vi "step2 SolveLowerLeftCornerPiece.vi"(8 "error in (no error)":errorcluster, 10 "operation queue":refnum<queue>, 11 "cube in":T1) -> (0 "error out":errorcluster, 2 "operation queue out":refnum<queue>, 3 "cube out":T1)   [LabVIEW 2011]
doc: "Rotate cube as necessary so that the top middle piece matches the desired start colour.\n\nNo transformations are done in this VI, the operations are loaded on the the operation queue bus."
uses:
  Typedef/cube.ctl
  Typedef/face.ctl
  Typedef/main state.ctl
  Typedef/operation.ctl
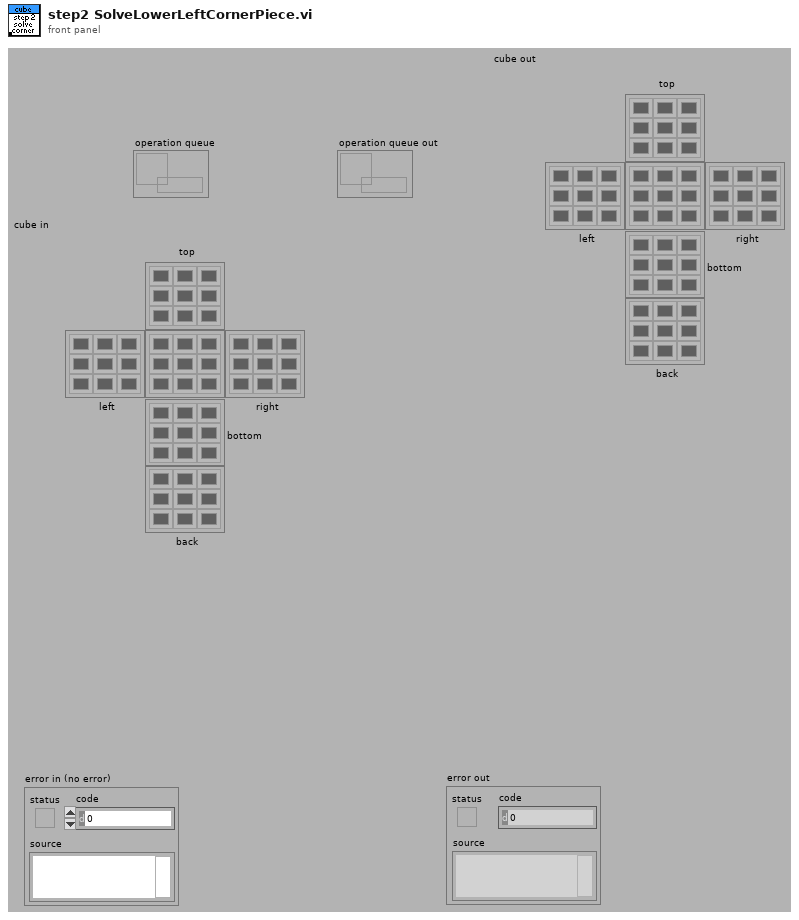
[diagram p1: front panel]
types:
  T1 = typedef "cube.ctl" = cluster{"top":T2, "left":T2, "right":T2, "bottom":T2, "back":T2, "front":T2}
  T2 = typedef "face.ctl" = u32[][]
  T3 = typedef "operation.ctl" = enum16{"nop", "T+", "T-", "F+", "F-", "L+", "L-", "R+", "R-", "B+", "B-", "<--", "-->", "^", "V"}
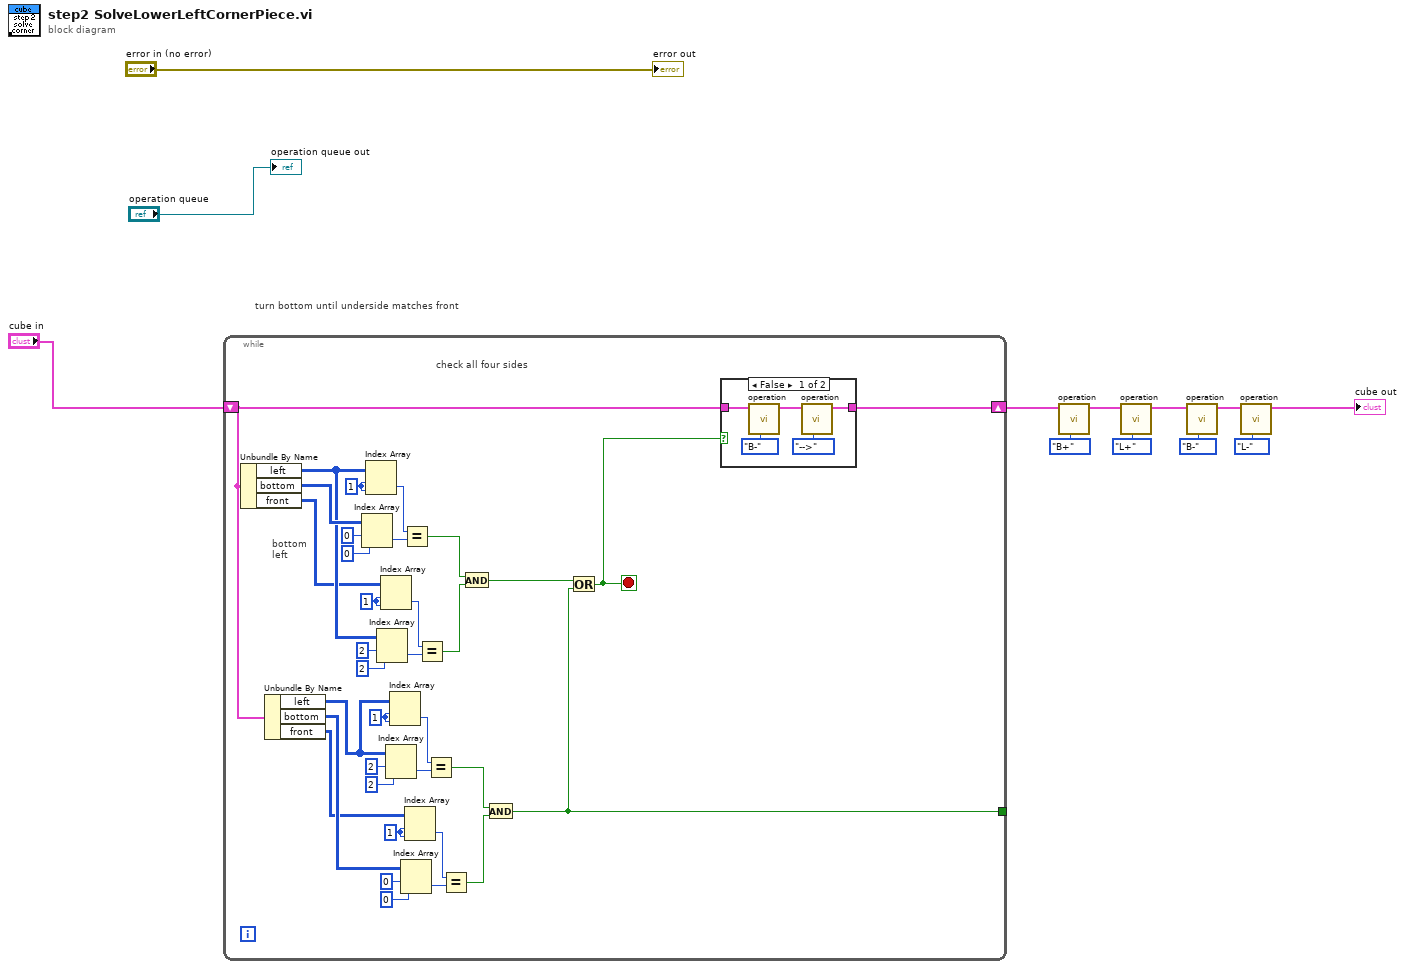
[diagram p0: block diagram]
diagram:
  # "turn bottom until underside matches front"
  n1 = while {
    shift-right: [w47] -> w5
    shift-left: "cube in" -> [w18]
    tunnel: [w13] -> _
    stop <- w14 stop-if-true
    w25 = 1 ("index (row)")
    w22 = 1 ("index (row)")
    w39 = 1 ("index (row)")
    w42 = 1 ("index (row)")
    # "bottom\nleft"
    # "check all four sides"
    n2 = Unbundle By Name(w18) -> ("left"=w35:T2, "bottom"=w43:T2, "front"=w34:T2)
    n3 = Unbundle By Name(w18) -> ("left"=w17:T2, "bottom"=w16:T2, "front"=w15:T2)
    n4 = Index Array(array=w43, index (row)=0, index (col)=0 ("index (row)")) -> (element=w44:u32)
    n5 = Index Array(array=w35, index (row)=w42, index (col)=w42) -> (element=w41:u32)
    n6 = Index Array(array=w35, index (row)=2, index (col)=2 ("index (row)")) -> (element=w38:u32)
    n7 = Index Array(array=w34, index (row)=w39, index (col)=w39) -> (element=w40:u32)
    n8 = Index Array(array=w17, index (row)=2, index (col)=2 ("index (row)")) -> (element=w21:u32)
    n9 = Index Array(array=w17, index (row)=w22, index (col)=w22) -> (element=w23:u32)
    n10 = Index Array(array=w16, index (row)=0, index (col)=0 ("index (row)")) -> (element=w26:u32)
    n11 = Equal?(x=w41, y=w44) -> (x = y?=w33:bool)
    n12 = Index Array(array=w15, index (row)=w25, index (col)=w25) -> (element=w24:u32)
    n13 = Equal?(x=w40, y=w38) -> (x = y?=w32:bool)
    n14 = Equal?(x=w23, y=w21) -> (x = y?=w29:bool)
    n15 = Equal?(x=w24, y=w26) -> (x = y?=w30:bool)
    n16 = And(x=w33, y=w32) -> (x .and. y?=w31:bool)
    n17 = And(x=w29, y=w30) -> (x .and. y?=w13:bool)
    n18 = Or(x=w31, y=w13) -> (x .or. y?=w14:bool)
    n19 = case shown="False" w14 {
      tunnel: w18 -> [w50 w53]
      tunnel: [w48 w53] -> w47
      frame False {
        n20 = call "operation.vi"("operation"=operation."B-", "cube in"=w50) -> ("cube out"=w49:T1)  [unwired: 8 in, 1 out]
        n21 = call "operation.vi"("operation"=operation."-->", "cube in"=w49) -> ("cube out"=w48:T1)  [unwired: 8 in, 1 out]
      }
      frame True {
      }
    }
  }
  n22 = call "operation.vi"("operation"=operation."B+", "cube in"=w5) -> ("cube out"=w4:T1)  [unwired: 8 in, 1 out]
  n23 = call "operation.vi"("operation"=operation."L+", "cube in"=w4) -> ("cube out"=w3:T1)  [unwired: 8 in, 1 out]
  n24 = call "operation.vi"("operation"=operation."B-", "cube in"=w3) -> ("cube out"=w2:T1)  [unwired: 8 in, 1 out]
  n25 = call "operation.vi"("operation"=operation."L-", "cube in"=w2) -> ("cube out"=→"cube out":T1)  [unwired: 8 in, 1 out]
  "error out" <- "error in (no error)"
  "operation queue out" <- "operation queue"
